vi "Cleanup.vi"(8 "error in":errorcluster, 11 "Philips Subpanel in":refnum<class "Flex UI Subpanel.lvclass">) -> (0 "error out":errorcluster)   [LabVIEW 2014, in "Flex UI Subpanel.lvclass"]
doc: "Cleans up after the UI.\n\nRuns EVEN IF an error has occurred upstream."
uses:
  Flex UI Subpanel.lvclass
  Flex UI Subpanel.lvclass/Flex UI Subpanel.ctl
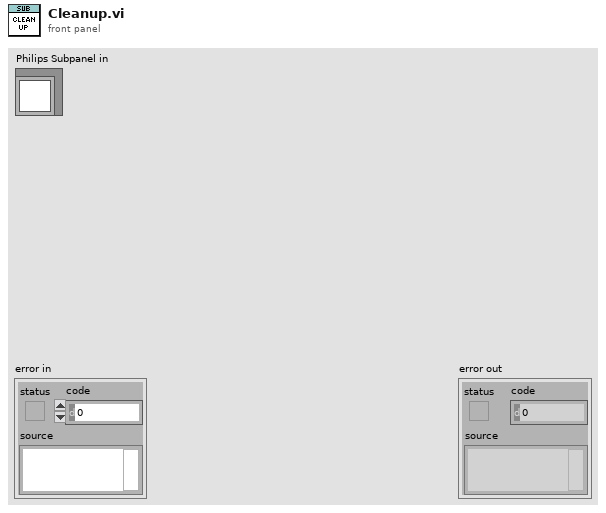
[diagram p1: front panel]
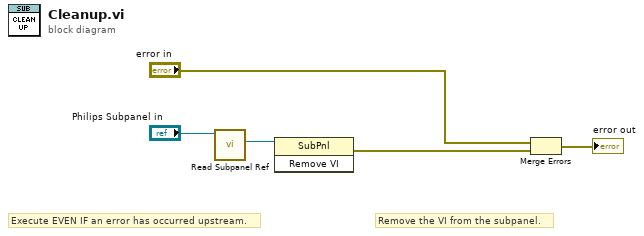
[diagram p0: block diagram]
diagram:
  # "Execute EVEN IF an error has occurred upstream."
  # "Remove the VI from the subpanel."
  n1 = call "Read Subpanel Ref.vi"("Philips Subpanel in"="Philips Subpanel in") -> ("Subpanel Ref"=w3:refnum<vi>)  [unwired: 9 in, 1 out]
  n2 = invoke class="SubPnl" method="Remove VI"(reference=w3) -> (error out=w4:errorcluster)  [unwired: 2 in, 2 out]
  n3 = Merge Errors("error in", w4) -> (→"error out":errorcluster)
